vi "Import Frames RTM.vi"(8 "error in":errorcluster, 11 "Node Ptr":u64 format="%.0x") -> (0 "error out":errorcluster)   [LabVIEW 2020, in "Communication Bus Template System Explorer.lvlib"]
doc: "This VI runs when the Import Frames run-time menu is chosen. It allows the user to import frames from the database associated with the port that will contain these frames."
uses:
  Communication Bus Template System Explorer.lvlib
  Shared/Constants.vi
  <vilib>/NI VeriStand/Custom Device API/Get Item Property (String).vi
  <vilib>/NI VeriStand/Custom Device API/Get Item Property (Path).vi
  Shared/Communication Bus Template Shared.lvlib
  <vilib>/NI VeriStand/Custom Device Tools/Custom Device Utility Library/Custom Device Utility Library.lvlib
  <vilib>/NI VeriStand/Custom Device API/Custom Device API.lvlib
  Scripting/Communication Bus Template Scripting.lvlib
  <vilib>/NI VeriStand/Custom Device API/Custom Device Channel Type.ctl
  <vilib>/NI VeriStand/Custom Device API/Custom Device Channel.ctl
  <vilib>/NI VeriStand/Custom Device Tools/Custom Device Utility Library/NI VeriStand - Search for Item by GUID.vi
  <vilib>/NI VeriStand/Custom Device Tools/Custom Device Utility Library/Search Direction.ctl
panel:
  in  "Select Frames":i32[](listbox)
  out "Database":string
  in  "Help":bool
  in  "Cancel":bool
  in  "OK":bool
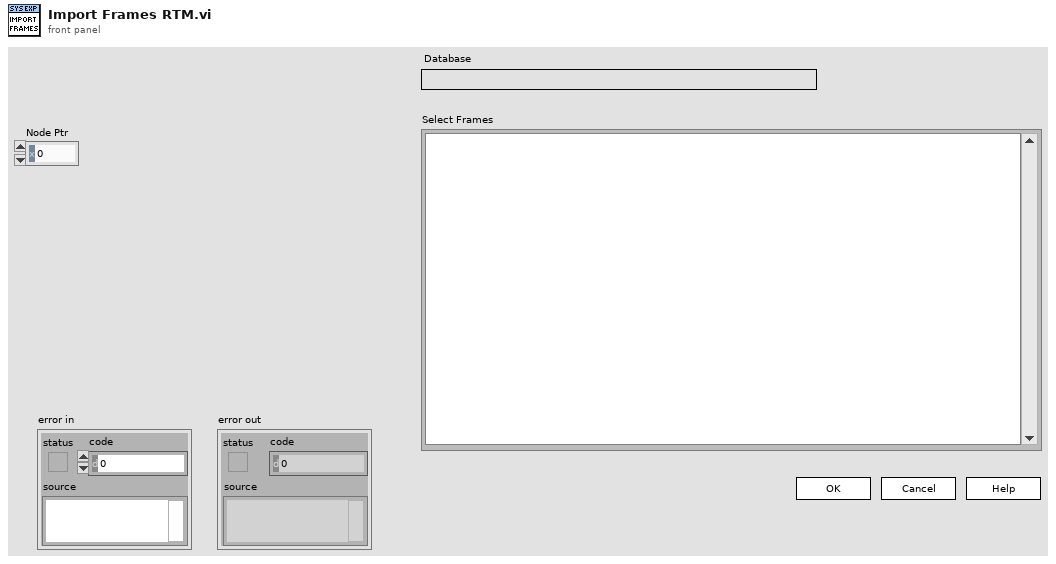
[diagram p1: front panel]
types:
  T1 = typedef "Custom Device Utility Library.lvlib/Search Direction.ctl" = enum16{"Down", "Up"}
  T2 = typedef "Custom Device API.lvlib/Custom Device Channel.ctl" = cluster{"Type":T3, "Units":string, "Default Value":dbl, "Faultable":bool, "Scalable":bool}
  T3 = typedef "Custom Device API.lvlib/Custom Device Channel Type.ctl" = enum16{"Input", "Output"}
  T4 = typedef "Custom Device API.lvlib/Custom Device Item Ref.ctl" = u64
  T5 = typedef "Communication Bus Template System Explorer.lvlib/Database.ctl" = cluster{"Baud Rate":u64, "Frames":cluster{"Name":string, "ID":i32}[]}
  T6 = cluster{"Channel":T2, "Node Ptr":u64, "Frames":cluster{"Name":string, "ID":i32}[]}
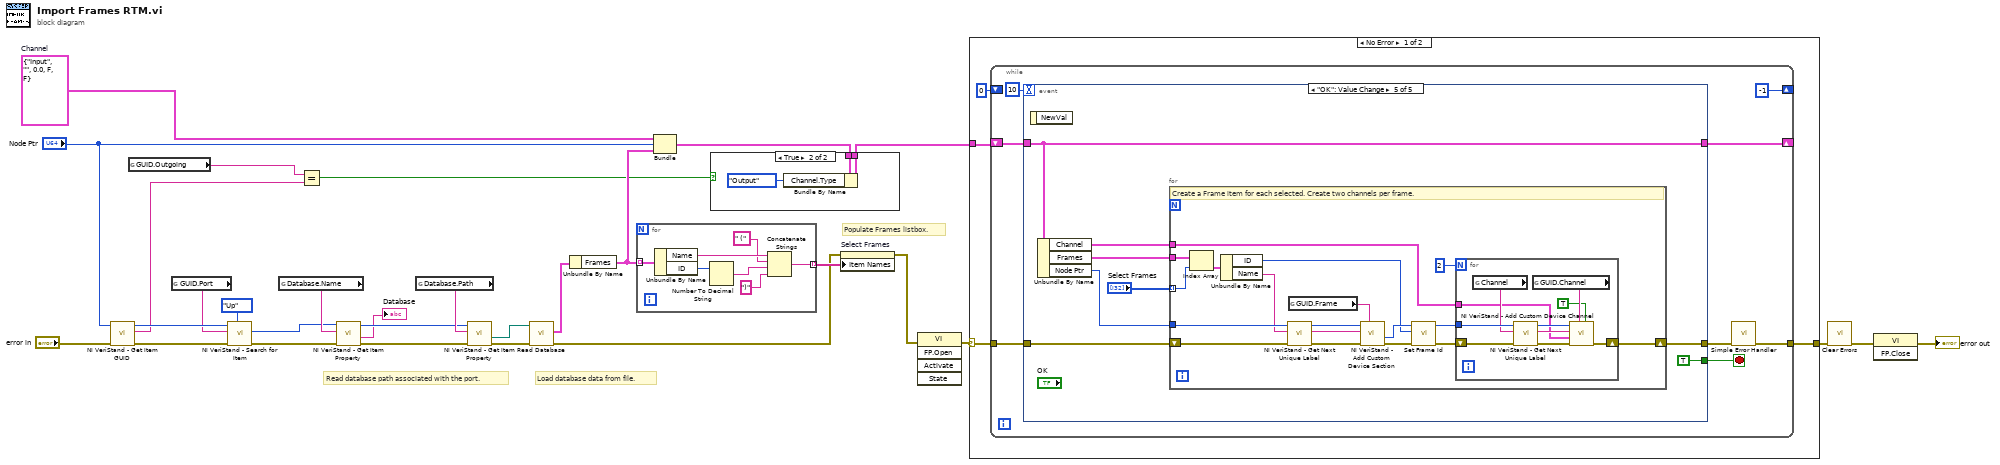
[diagram p0: block diagram]
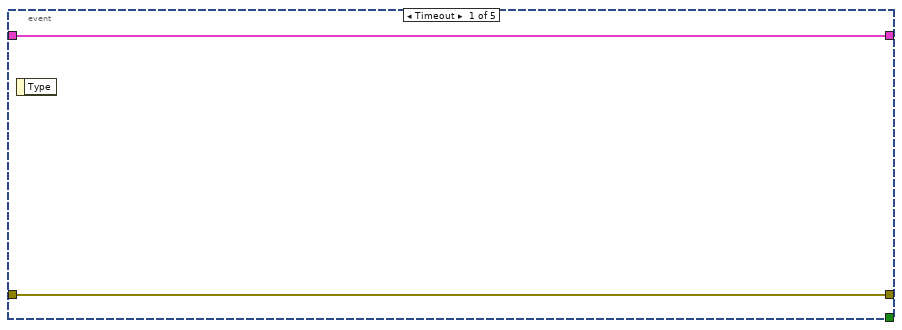
[diagram p3: hidden frame]
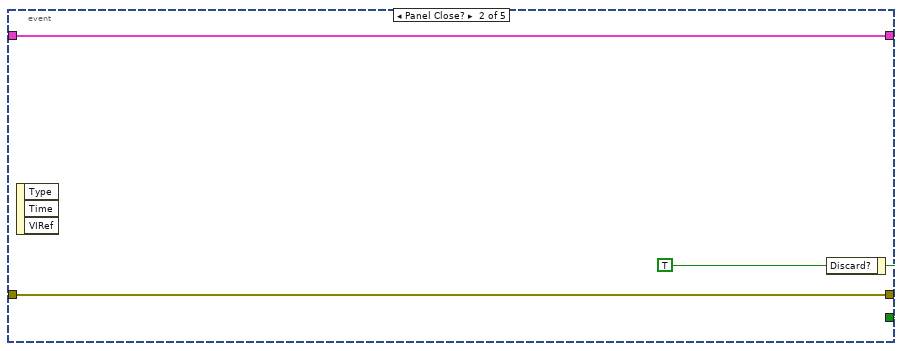
[diagram p4: hidden frame]
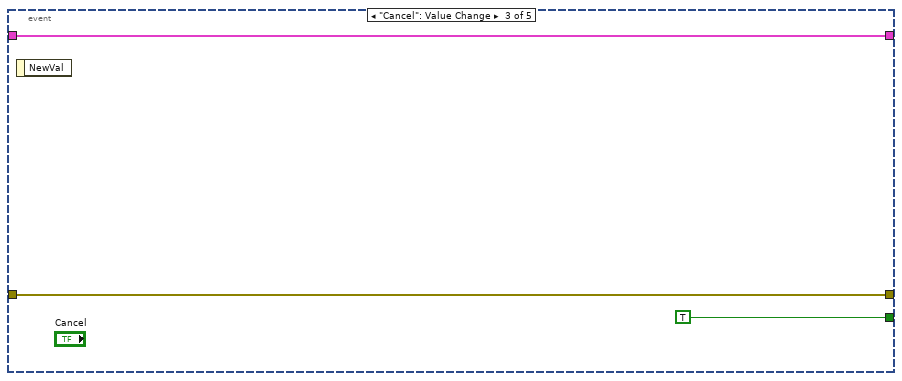
[diagram p5: hidden frame]
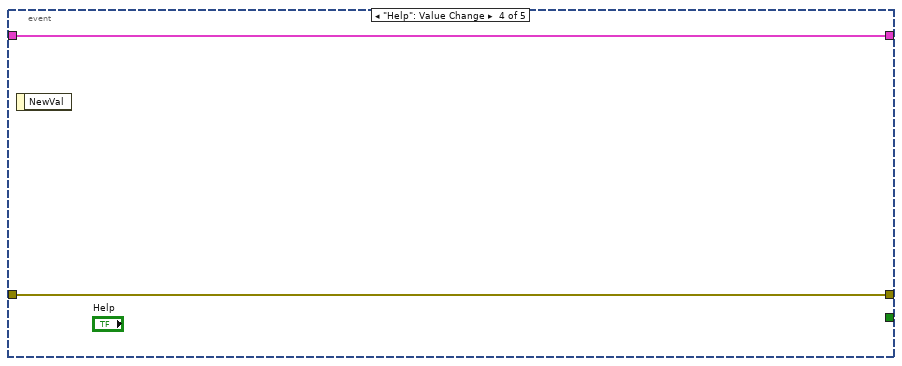
[diagram p6: hidden frame]
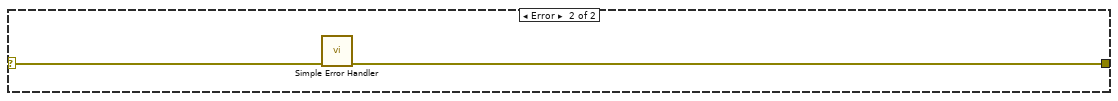
[diagram p7: hidden frame]
diagram:
  w8 = T2 {"Type"=enum."Input", "Units"="", "Default Value"=0.0, "Faultable"=FALSE, "Scalable"=FALSE}  # Channel
  # "Populate Frames listbox."
  # "Load database data from file."
  # "Read database path associated with the port."
  n1 = call <vilib>:"NI VeriStand - Get Item GUID.vi"("error in (no error)"="error in", "Item Ref in"="Node Ptr") -> ("error out"=w11:errorcluster, "GUID"=w4:string, "Item Ref out"=w9:T4)  [unwired: 7 in]
  n2 = global read "Constants.vi" "GUID.Outgoing"() -> (w5:string)
  n3 = global read "Constants.vi" "GUID.Port"() -> (w2:string)
  n4 = call-poly <vilib>:"NI VeriStand - Search for Item.vi"("Direction (Down)"=Search_Direction."Up", "error in"=w11, "Item GUID"=w2, "Section Ref in"=w9) -> ("error out"=w14:errorcluster, "Item Ref"=w13:T4)  [unwired: 4 in, 2 out]
  n5 = global read "Constants.vi" "Database.Name"() -> (w21:string)
  n6 = Equal?(x=w5, y=w4) -> (x = y?=w3:bool)
  n7 = call-poly <vilib>:"NI VeriStand - Get Item Property.vi"("error in (no error)"=w14, "Property Name"=w21, "Item Ref in"=w13) -> ("error out"=w20:errorcluster, "Value"=→"Database":string, "Item Ref out"=w19:T4)  [unwired: 5 in, 1 out]
  n8 = global read "Constants.vi" "Database.Path"() -> (w27:string)
  n9 = call-poly <vilib>:"NI VeriStand - Get Item Property.vi"("error in (no error)"=w20, "Property Name"=w27, "Item Ref in"=w19) -> ("error out"=w26:errorcluster, "Value"=w17:path)  [unwired: 5 in, 2 out]
  n10 = call "Read Database.vi"("error in"=w26, "Path"=w17) -> ("error out"=w22:errorcluster, "Database"=w25:T5)  [unwired: 8 in]
  n11 = Unbundle By Name(w25) -> ("Frames"=w23:cluster{"Name":string, "ID":i32}[])
  n12 = for {
    tunnel: w23 -> [w37] mode=indexing
    tunnel: [w31] -> w24 mode=indexing
    n13 = Unbundle By Name(w37) -> ("Name"=w35:string, "ID"=w36:i32)
    n14 = Number To Decimal String(number=w36) -> (decimal integer string=w33:string)  [unwired: 1 in]
    n15 = Concatenate Strings(w35, " (" ("string"), w33, ")" ("string")) -> (w31:string)
  }
  n16 = Bundle("Channel"=w8, "Node Ptr"="Node Ptr", "Frames"=w23) -> (w7:T6)  [unwired: 1 in]
  n17 = case shown="True" w3 {
    tunnel: w7 -> [w38 w40]
    tunnel: [w38 w39] -> w6
    frame False {
    }
    frame True {
      n18 = Bundle By Name(cluster=w40, "Channel.Type"=Custom_Device_Channel_Type."Output") -> (w39:T6)
    }
  }
  n19 = property on="Select Frames" class="LstBox (strict)"(error in=w22, "Item Names"=w24) -> (error out=w15:errorcluster)  [unwired: 1 in, 1 out]
  n20 = invoke class="VI" method="FP.Open"(error in=w15) -> (error out=w16:errorcluster)  [unwired: 4 in, 4 out]
  n21 = case shown="No Error" w16 {
    selector: w16 -> [w45 w101]
    tunnel: [w44 w100] -> w30
    tunnel: w6 -> [w42 _]
    frame No Error {
      n22 = while {
        tunnel: w45 -> [w53]
        tunnel: [w51] -> w44
        shift-right: [-1] -> _
        shift-left: 0 -> [_]
        shift-right: [w47] -> _
        shift-left: w42 -> [w48]
        stop <- w50 stop-if-true
        n23 = event shown="[4] \"OK\": Value Change" {
          selector: _ -> [_ _ _ _ _]
          dyn-events: _ -> [_ _ _ _ _]
          timeout: 10 -> [_ _ _ _ _]
          tunnel: [w55 w58 w60 w63 w67] -> w52
          tunnel: w53 -> [w55 w58 w60 w63 w70]
          tunnel: [_ w57 TRUE ("Discard?") _ TRUE ("Discard?")] -> w50
          tunnel: w48 -> [w54 w56 w59 w62 w69]
          tunnel: [w54 w56 w59 w62 w69] -> w47
          event Timeout {
            n24 = event-data() -> ()  [unwired: 1 in, 1 out]
          }
          event Panel Close? {
            w57 = TRUE ("Discard?")
            n25 = event-data() -> ()  [unwired: 1 in, 3 out]
            n26 = event-data("Discard?"=w57) -> ()  [unwired: 1 in, 1 out]
          }
          event "Cancel": Value Change {
            n27 = event-data() -> ()  [unwired: 1 in, 1 out]
          }
          event "Help": Value Change {
            n28 = event-data() -> ()  [unwired: 1 in, 1 out]
          }
          event "OK": Value Change {
            n29 = event-data() -> ()  [unwired: 1 in, 1 out]
            n30 = Unbundle By Name(w69) -> ("Channel"=w64:T2, "Frames"=w66:cluster{"Name":string, "ID":i32}[], "Node Ptr"=w68:u64)
            n31 = for {
              tunnel: w68 -> [w84]
              shift-right: [w72] -> w67
              shift-left: w70 -> [w87]
              tunnel: w66 -> [w81]
              tunnel: "Select Frames" -> [w80] mode=indexing
              tunnel: w64 -> [w73]
              # "Create a Frame item for each selected. Create two channels per frame."
              n32 = Index Array(array=w81, index=w80) -> (element=w79:cluster{"Name":string, "ID":i32})
              n33 = Unbundle By Name(w79) -> ("ID"=w77:i32, "Name"=w78:string)
              n34 = call <vilib>:"NI VeriStand - Get Next Unique Label.vi"("error in (no error)"=w87, "Label"=w78, "Parent Ref in"=w84) -> ("error out"=w88:errorcluster, "Label out"=w85:string, "Parent Ref dup"=w86:T4)  [unwired: 5 in, 1 out]
              n35 = global read "Constants.vi" "GUID.Frame"() -> (w89:string)
              n36 = call <vilib>:"NI VeriStand - Add Custom Device Section.vi"("GUID (Default Section)"=w89, "error in (no error)"=w88, "Section Name"=w85, "Parent Ref in"=w86) -> ("error out"=w83:errorcluster, "Section Ptr"=w82:T4)  [unwired: 4 in, 2 out]
              n37 = call "Set Frame Id.vi"("error in"=w83, "ID"=w77, "Node Ptr"=w82) -> ("error out"=w75:errorcluster, "Node Ptr out"=w74:T4)  [unwired: 7 in]
              n38 = for {
                N: 2 -> [_]
                shift-right: [w98] -> w72
                shift-left: w75 -> [w99]
                tunnel: w74 -> [w94]
                tunnel: w73 -> [w91]
                n39 = global read "Constants.vi" "Channel"() -> (w92:string)
                n40 = call <vilib>:"NI VeriStand - Get Next Unique Label.vi"("error in (no error)"=w99, "Label"=w92, "Parent Ref in"=w94) -> ("error out"=w96:errorcluster, "Label out"=w97:string, "Parent Ref dup"=w95:T4)  [unwired: 5 in, 1 out]
                n41 = global read "Constants.vi" "GUID.Channel"() -> (w93:string)
                n42 = call <vilib>:"NI VeriStand - Add Custom Device Channel.vi"("Highlight? (F)"=TRUE, "GUID (Default Channel)"=w93, "error in (no error)"=w96, "Channel"=w91, "Channel Name"=w97, "Parent Ref in"=w95) -> ("error out"=w98:errorcluster)  [unwired: 2 in, 3 out]
              }
            }
          }
        }
        n43 = call <vilib>:"Simple Error Handler.vi"("error in (no error)"=w52) -> ("error out"=w51:errorcluster)  [unwired: 4 in, 4 out]
      }
    }
    frame Error {
      n44 = call <vilib>:"Simple Error Handler.vi"("error in (no error)"=w101) -> ("error out"=w100:errorcluster)  [unwired: 4 in, 4 out]
    }
  }
  n45 = call <vilib>:"Clear Errors.vi"("error in (no error)"=w30) -> ("error out"=w29:errorcluster)  [unwired: 5 in, 1 out]
  n46 = invoke class="VI" method="FP.Close"(error in=w29) -> (error out=→"error out":errorcluster)  [unwired: 2 in, 2 out]
